vi "rename channel.vi"(8 "error in":errorcluster, 9 "new name":string, 10 "old name":string, 11 "Tagbus PID Module configuration in":refnum<class "Tagbus PID Module configuration.lvclass">) -> (0 "error out":errorcluster, 3 "Tagbus PID Module configuration out":refnum<class "Tagbus PID Module configuration.lvclass">)   [LabVIEW 2014]
uses:
  <vilib>/NI/Tag Bus/tag/tag descriptor.lvclass
  Tagbus PID Module configuration.lvclass
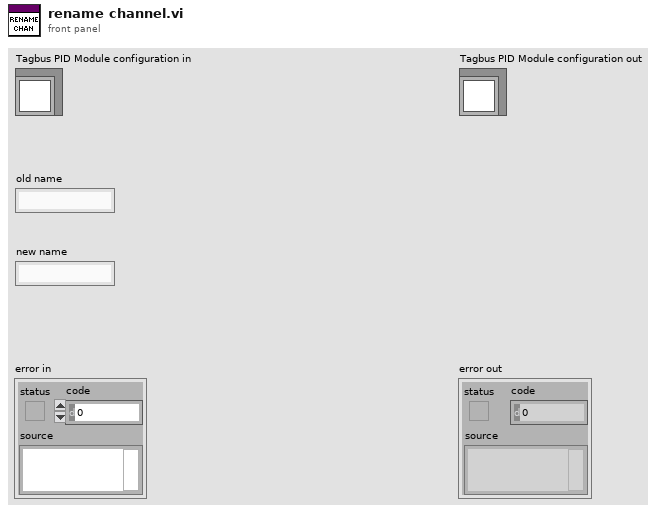
[diagram p1: front panel]
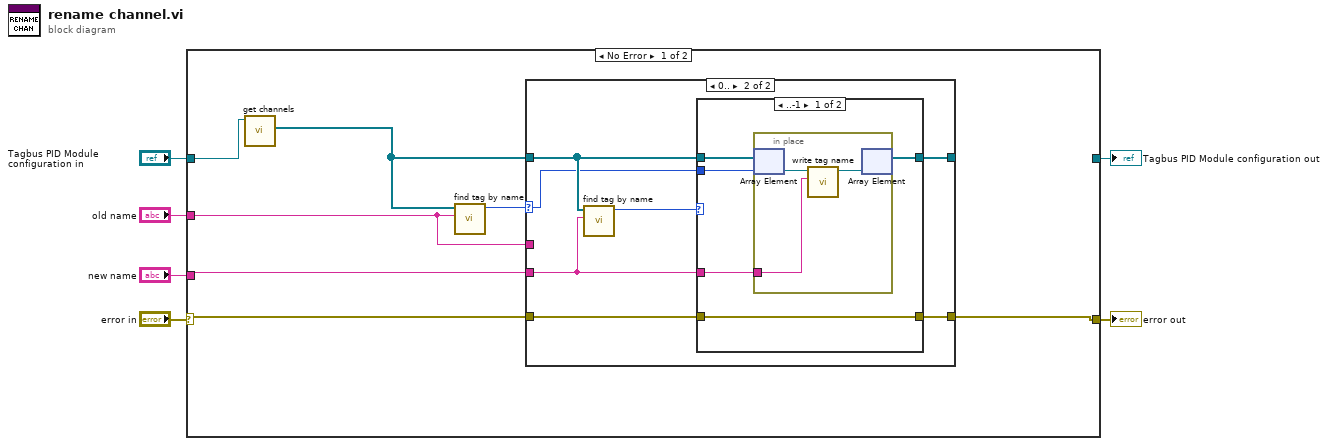
[diagram p0: block diagram]
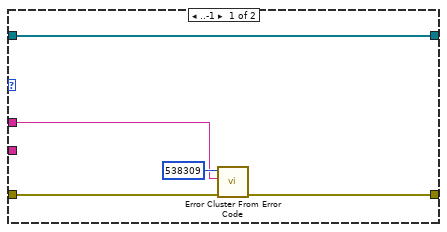
[diagram p2: hidden frame]
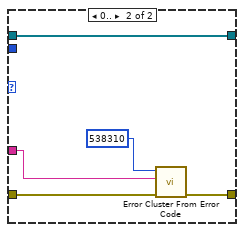
[diagram p3: hidden frame]
diagram:
  n1 = case shown="No Error" "error in" {
    selector: "error in" -> [w10 w40]
    tunnel: "new name" -> [w13 _]
    tunnel: "Tagbus PID Module configuration in" -> [w9 w39]
    tunnel: [_ w39] -> w4
    tunnel: [w12 w40] -> w3
    tunnel: "old name" -> [w11 _]
    frame No Error {
      n2 = call-dynamic "get channels.vi"("Tagbus PID Module configuration in"=w9) -> ("channels"=w7:refnum<class "TBM channel.lvclass">[])  [unwired: 9 in, 1 out]
      n3 = call <vilib>:"find tag by name.vi"("name"=w11, "tags in"=w7) -> ("index"=w8:i32)  [unwired: 9 in]
      n4 = case shown="0.." w8 {
        selector: w8 -> [_ w19]
        tunnel: w7 -> [w15 w24]
        tunnel: w11 -> [w17 _]
        tunnel: [w16 w20] -> w12
        tunnel: [w15 w25] -> _
        tunnel: w10 -> [w14 w21]
        tunnel: w13 -> [_ w23]
        frame ..-1 {
          n5 = call <vilib>:"Error Cluster From Error Code.vi"("error in (no error)"=w14, "error message (\"\")"=w17, "error code (0)"=538309) -> ("error out"=w16:errorcluster)  [unwired: 6 in]
        }
        frame 0.. {
          n6 = call <vilib>:"find tag by name.vi"("name"=w23, "tags in"=w24) -> ("index"=w22:i32)  [unwired: 9 in]
          n7 = case shown="..-1" w22 {
            tunnel: [w30 w38] -> w25
            tunnel: w19 -> [w29 _]
            tunnel: w24 -> [w28 w38]
            tunnel: w23 -> [w27 w34]
            tunnel: w21 -> [w26 w36]
            tunnel: [w26 w37] -> w20
            frame ..-1 {
              n8 = in-place {
                in-place-border: w27 -> [w31]
                n9 = in-place-array #1(w28, w29) -> (w33:refnum<class "TBM channel.lvclass">)
                n10 = call <vilib>:"write tag name.vi"("name"=w31, "system tag in"=w33) -> ("system tag out"=w32:refnum<class "TBM channel.lvclass">)  [unwired: 8 in, 1 out]
                n11 = in-place-array #1(w32) -> (w30:refnum<class "TBM channel.lvclass">[])  [unwired: 1 out]
              }
            }
            frame 0.. {
              n12 = call <vilib>:"Error Cluster From Error Code.vi"("error in (no error)"=w36, "error message (\"\")"=w34, "error code (0)"=538310) -> ("error out"=w37:errorcluster)  [unwired: 6 in]
            }
          }
        }
      }
    }
    frame Error {
    }
  }
  "error out" <- w3
  "Tagbus PID Module configuration out" <- w4
